vi "XML ( Delete Node Value Single Input ).vi"(8 "error in (no error)":errorcluster, 9 "Child_Node":string, 10 "Parent_Node":string, 11 "XML in":refnum<class "XML.lvclass">) -> (0 "error out":errorcluster, 3 "XML out":refnum<class "XML.lvclass">)   [LabVIEW 2018, in "XML.lvlib" / "XML.lvclass"]
uses:
  XML.lvclass
  XML.lvclass/XML.ctl
  <vilib>/xml/Close Reference(Node).vi
  <vilib>/xml/NI_XML.lvlib
  <resource>/objmgr/DOMUserDefRef.rc
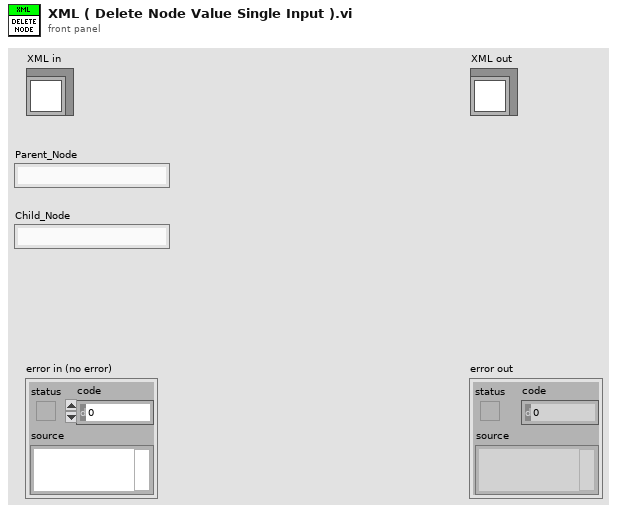
[diagram p1: front panel]
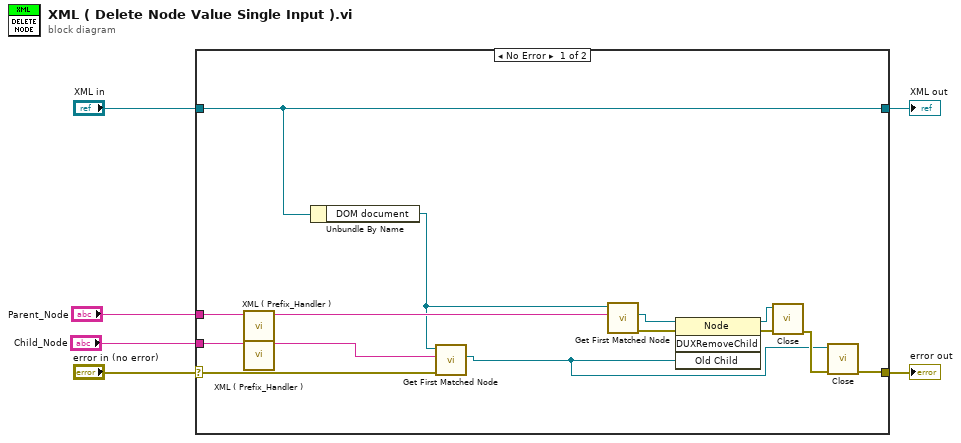
[diagram p0: block diagram]
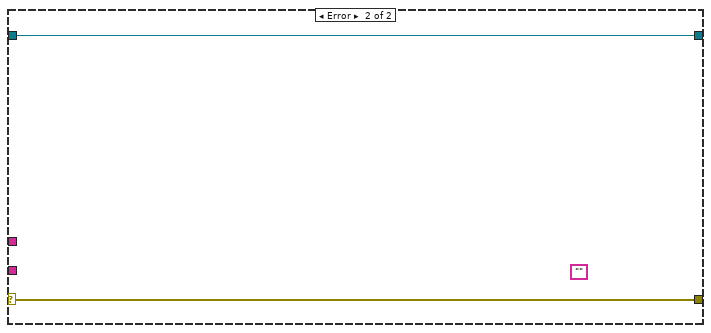
[diagram p2: hidden frame]
diagram:
  n1 = case shown="No Error" "error in (no error)" {
    selector: "error in (no error)" -> [w10 w22]
    tunnel: [w9 w22] -> w5
    tunnel: [w20 w21] -> w3
    tunnel: "XML in" -> [w20 w21]
    tunnel: "Parent_Node" -> [w15 _]
    tunnel: "Child_Node" -> [w13 _]
    frame No Error {
      n2 = call "XML ( Prefix_Handler ).vi"("input string"=w15) -> ("result string"=w14:string)  [unwired: 10 in]
      n3 = call "XML ( Prefix_Handler ).vi"("input string"=w13) -> ("result string"=w11:string)  [unwired: 10 in]
      n4 = Unbundle By Name(w20) -> ("DOM document"=w12:refnum<k20>)
      n5 = call <vilib>:"Get First Matched Node.vi"("error in (no error)"=w10, "XPath expression"=w11, "node in"=w12) -> ("node result"=w7:refnum<k20>)  [unwired: 6 in, 2 out]
      n6 = call <vilib>:"Get First Matched Node.vi"("XPath expression"=w14, "node in"=w12) -> ("error out"=w18:errorcluster, "node result"=w19:refnum<k20>)  [unwired: 7 in, 1 out]
      n7 = invoke class="Node" method="DUXRemoveChild"(reference=w19, error in=w18, "Old Child"=w7) -> (reference out=w16:refnum<k20>, error out=w17:errorcluster)  [unwired: 1 in, 2 out]
      n8 = call-poly <vilib>:"Close.vi"("error in (no error)"=w17, "node"=w16) -> ("error out"=w8:errorcluster)  [unwired: 7 in]
      n9 = call-poly <vilib>:"Close.vi"("error in (no error)"=w8, "node"=w7) -> ("error out"=w9:errorcluster)  [unwired: 7 in]
    }
    frame Error {
      (unwired) ""
    }
  }
  "error out" <- w5
  "XML out" <- w3
